vi "Get Available MetaData Channels.vi"(8 "error in (no error)":errorcluster, 10 "Command":refnum<vi>, 11 "Item Ref in":T1 format="%.0x") -> (0 "error out":errorcluster, 3 "Item Ref out":T1 format="%.0x")   [LabVIEW 2018, in "Instrument Addon System Explorer.lvlib"]
uses:
  Instrument Addon System Explorer.lvlib
  <vilib>/NI Veristand/Custom Device API/Custom Device Item Ref.ctl
  Addon Shared/SubVIs/Constants.vi
  <vilib>/NI Veristand/Custom Device API/Get Item Property (String).vi
  <vilib>/NI VeriStand/Custom Device API/Custom Device API.lvlib
  Addon Shared/Instrument Addon Shared.lvlib
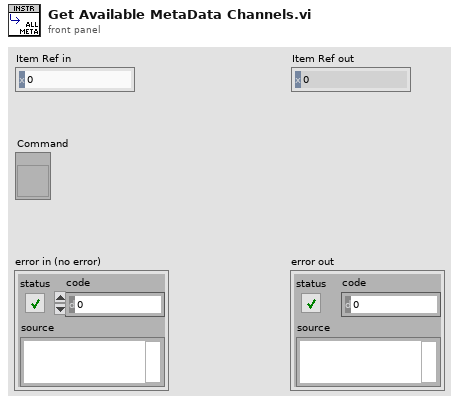
[diagram p1: front panel]
types:
  T1 = typedef "Custom Device API.lvlib/Custom Device Item Ref.ctl" = u64
  T2 = typedef "Custom Device API.lvlib/Custom Device Item Info.ctl" = cluster{"Name":string, "Is Channel":bool, "GUID":string, "Is Waveform":bool}
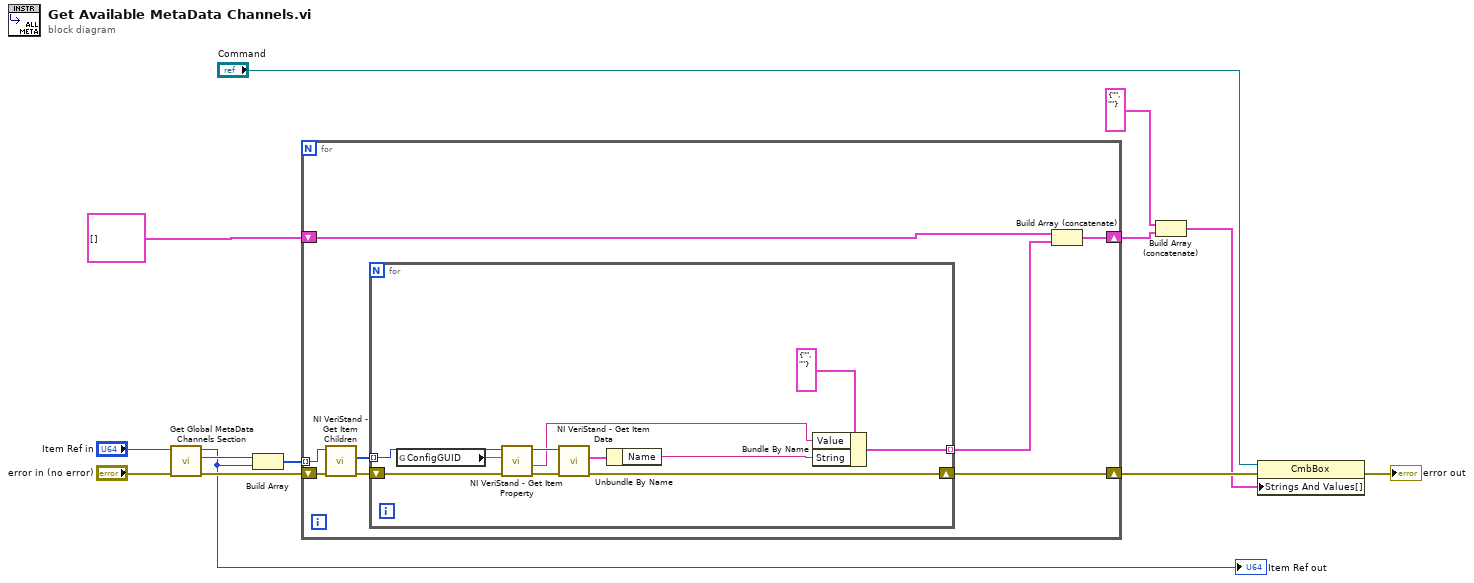
[diagram p0: block diagram]
diagram:
  n1 = call "Get Global MetaData Channels Section.vi"("error in (no error)"="error in (no error)", "Item Ref in"="Item Ref in") -> ("error out"=w13:errorcluster, "Item Ref"=w10:T1, "Item Ref out"=w8:T1)  [unwired: 7 in]
  "Item Ref out" <- w8
  n2 = Build Array(w10, w8) -> (w12:T1[])
  n3 = for {
    tunnel: w12 -> [w17] mode=indexing
    shift-right: [w21] -> w6
    shift-left: w13 -> [w18]
    shift-right: [w15] -> w2
    shift-left: cluster{"String":string, "Value":string}[] [] ("Strings And Values []") -> [w16]
    n4 = call <vilib>:"NI VeriStand - Get Item Children.vi"("error in (no error)"=w18, "Item Ref in"=w17) -> ("error out"=w19:errorcluster, "Child Refs"=w20:T1[])  [unwired: 6 in, 2 out]
    n5 = for {
      tunnel: w20 -> [w31] mode=indexing
      shift-right: [w30] -> w21
      shift-left: w19 -> [w27]
      tunnel: [w29] -> w14 mode=indexing
      n6 = global read "Constants.vi" "ConfigGUID"() -> (w25:string)
      n7 = call-poly <vilib>:"NI VeriStand - Get Item Property.vi"("error in (no error)"=w27, "Property Name"=w25, "Item Ref in"=w31) -> ("error out"=w26:errorcluster, "Value"=w22:string, "Item Ref out"=w28:T1)  [unwired: 5 in, 1 out]
      n8 = call <vilib>:"NI VeriStand - Get Item Data.vi"("error in (no error)"=w26, "Item Ref in"=w28) -> ("error out"=w30:errorcluster, "Item Info"=w32:T2)  [unwired: 8 out]
      n9 = Unbundle By Name(w32) -> ("Name"=w23:string)
      n10 = Bundle By Name(cluster=cluster{"String":string, "Value":string} {"String"="", "Value"=""}, "Value"=w22, "String"=w23) -> (w29:cluster{"String":string, "Value":string})
    }
    n11 = Build Array (concatenate)(w16, w14) -> (w15:cluster{"String":string, "Value":string}[])
  }
  n12 = Build Array (concatenate)(cluster{"String":string, "Value":string} {"String"="", "Value"=""}, w2) -> (w1:cluster{"String":string, "Value":string}[])
  n13 = property class="CmbBox"(reference="Command", error in=w6, "Strings And Values[]"=w1) -> (error out=→"error out":errorcluster)  [unwired: 1 out]
